vi "Delete Front Panel Controls.vi"(8 "error in (no error)":errorcluster, 11 "vi reference in":refnum<vi>) -> (0 "error out":errorcluster, 3 "vi reference out":refnum<vi>)   [LabVIEW 2019, in "gRPC Template Creation Utility.lvlib"]
uses:
  gRPC Template Creation Utility.lvlib
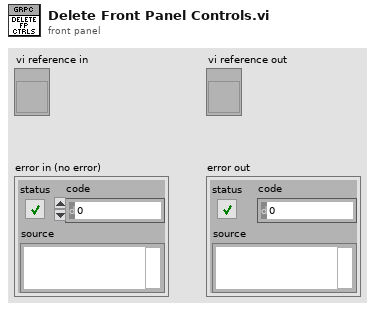
[diagram p1: front panel]
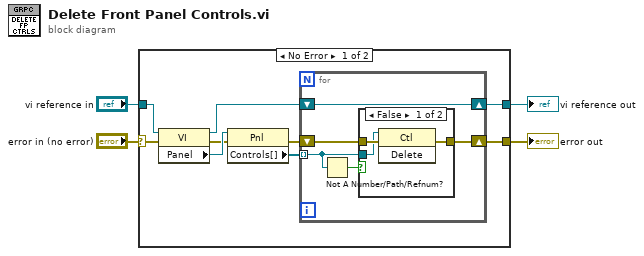
[diagram p0: block diagram]
diagram:
  n1 = case shown="No Error" "error in (no error)" {
    selector: "error in (no error)" -> [w13 w24]
    tunnel: [w9 w23] -> w1
    tunnel: [w11 w24] -> w3
    tunnel: "vi reference in" -> [w8 w23]
    frame No Error {
      n2 = property class="VI"(reference=w8, error in=w13) -> (reference out=w10:refnum<vi>, error out=w6:errorcluster, "Panel"=w12:refnum<vi>)
      n3 = property class="Pnl"(reference=w12, error in=w6) -> (error out=w5:errorcluster, "Controls[]"=w7:refnum<vi>[])  [unwired: 1 out]
      n4 = for {
        tunnel: w7 -> [w14] mode=indexing
        shift-right: [w18] -> w11
        shift-left: w5 -> [w15]
        shift-right: [w17] -> w9
        shift-left: w10 -> [w17]
        n5 = Not A Number/Path/Refnum?(number/path/refnum=w14) -> (NaN/Path/Refnum?=w16:bool)
        n6 = case shown="False" w16 {
          tunnel: [w21 w22] -> w18
          tunnel: w15 -> [w20 w22]
          tunnel: w14 -> [w19 _]
          frame False {
            n7 = invoke class="Ctl" method="Delete"(reference=w19, error in=w20) -> (error out=w21:errorcluster)  [unwired: 1 in, 2 out]
          }
          frame True {
          }
        }
      }
    }
    frame Error {
    }
  }
  "error out" <- w3
  "vi reference out" <- w1
